vi "GIP CAN Wrapper.vi"(6 "Signal Write":dbl, 7 "States":T1, 8 "error in":errorcluster, 9 "Setting":T2={"Termination"=1, "Baud Rate"=125000, "Interface"="CAN1", "XNET Database"="can_messages_818", "ECU"="GIP\ncan_messages_818"} {"Termination" items=["Off", "On"]}, 10 "Tx Signal In":string="\"GIP_TestMode.GIP_TestModeFlag\"", 11 "Rx Signal In":string="\"GIP_Status.GIP_State\"") -> (0 "error out":errorcluster={"status"=TRUE, "code"=-1074384711, "source"="XNET Create Session (Signal Input Single-point).vi:6590001<APPEND>\n\n<b>Complete call chain:</b>\r\n     XNET Create Session (Signal Input Single-point).vi:6590001\r\n     CAN GIP.lvlib:GIP CAN Wrapper.vi"}, 1 "Tx Sigs":refnum<k21>[](array[refnum]), 2 "Rx Sigs":refnum<k21>[](array[refnum]), 3 "Signal out":dbl=nan)   [LabVIEW 2021, in "CAN GIP.lvlib"]
uses:
  CAN GIP.lvlib
  Private Controls/Setting.ctl
  Private Controls/CAN States.ctl
  Private Controls/Local Variables.ctl
  <vilib>/JDP Science/JSONtext/Next JSON Value.vi
  <vilib>/JDP Science/JSONtext/String Subset.vi
  <vilib>/JDP Science/JSONtext/Parsing/Advance past next JSON Value (inlined COPY).vi
  <vilib>/JDP Science/JSONtext/Parsing/Advance past whitespace.vi
  <vilib>/JDP Science/JSONtext/Parsing/Advance past String.vi
  <vilib>/JDP Science/JSONtext/Parsing/Advance past Number.vi
  <vilib>/JDP Science/JSONtext/Parsing/Advance past Line Ending.vi
  <vilib>/xnet/xnet.llb/XNET Create Session (Signal Input Single-point).vi
  <vilib>/xnet/xnet.llb/XNET Create Session (Signal Output Single-point).vi
  <vilib>/xnet/xnet.llb/XNET Read (Signal Single-point).vi
  <vilib>/JDP Science/JSONtext/Parsing/Parse Full Path or Item Name.vi
  <vilib>/JDP Science/JSONtext/Parsing/Advance past Array.vi
  <vilib>/JDP Science/JSONtext/Parsing/Advance past Object.vi
  <vilib>/JDP Science/JSONtext/support/Error Cluster From Code.vi
  <vilib>/JDP Science/JSONtext/Offset/Find Item Locations by Path.vi
  <vilib>/xnet/xnet.llb/XNET Write (Signal Single-point).vi
  <resource>/objmgr/xnet.rc
  <vilib>/JDP Science/JSONtext/JSONtext.lvlib
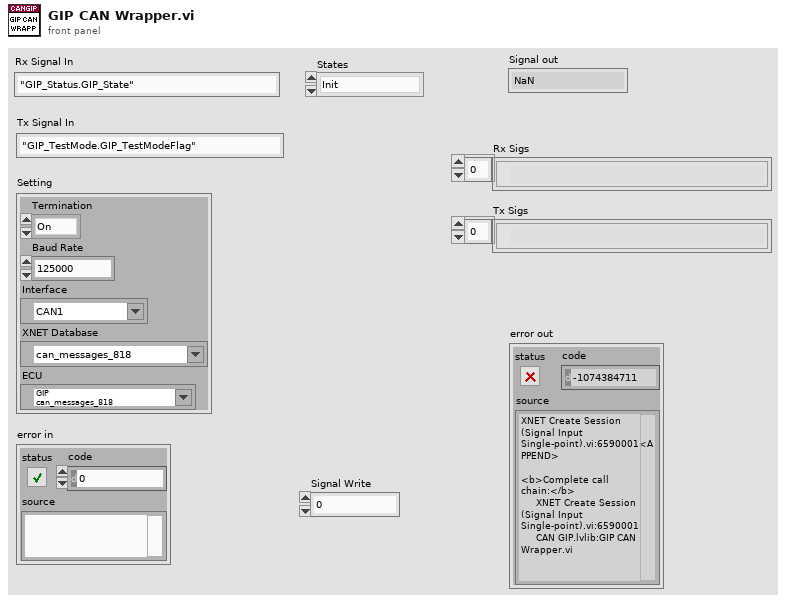
[diagram p1: front panel]
types:
  T1 = typedef "CAN GIP.lvlib/CAN States.ctl" = enum16{"Init", "Config", "Read Signals", "Write Signals", "Close"}
  T2 = typedef "CAN GIP.lvlib/Setting.ctl" = cluster{"Termination":u32, "Baud Rate":u64, "Interface":refnum<k21>, "XNET Database":refnum<k21>, "ECU":refnum<k21>}
  T3 = typedef "CAN GIP.lvlib/Local Variables.ctl" = cluster{"Rx session":refnum<k21>, "Tx session":refnum<k21>, "Tx Data":dbl[], "JSON":string}
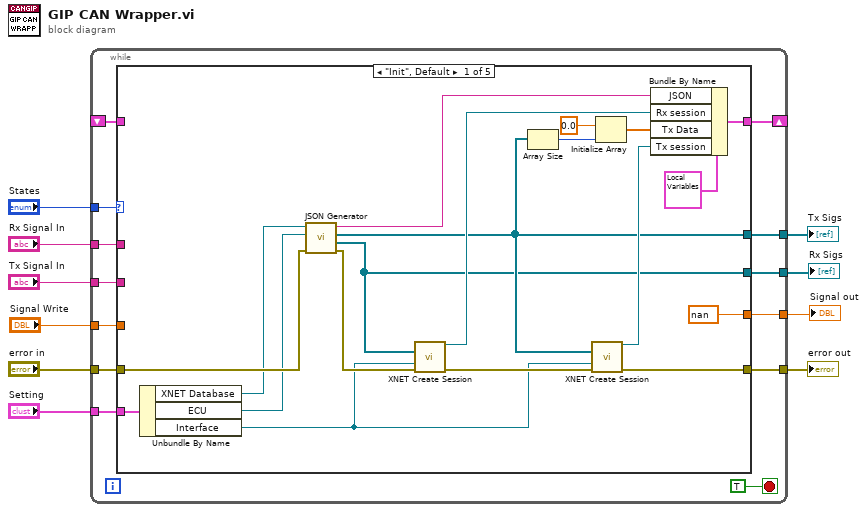
[diagram p0: block diagram]
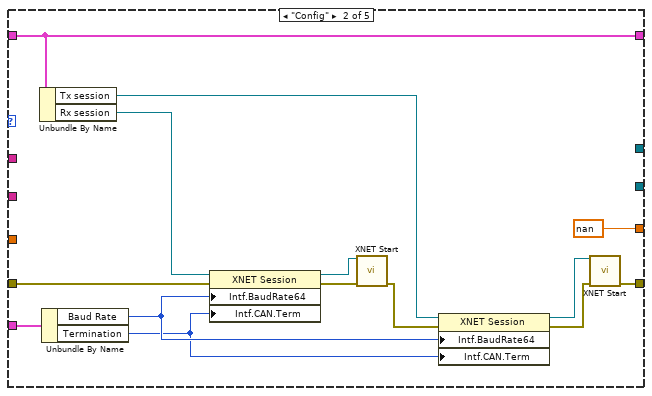
[diagram p2: hidden frame]
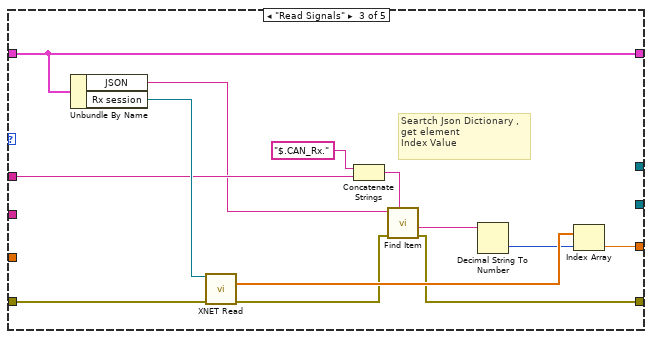
[diagram p3: hidden frame]
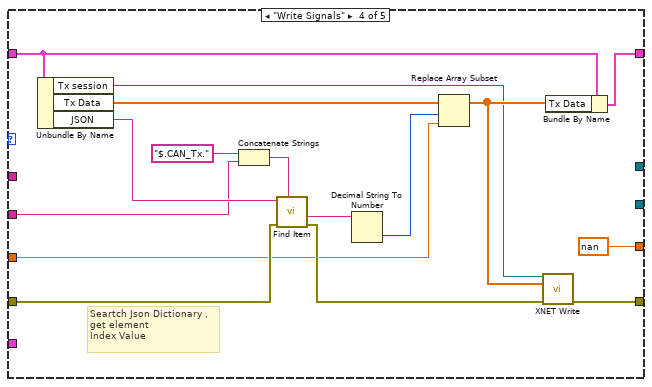
[diagram p4: hidden frame]
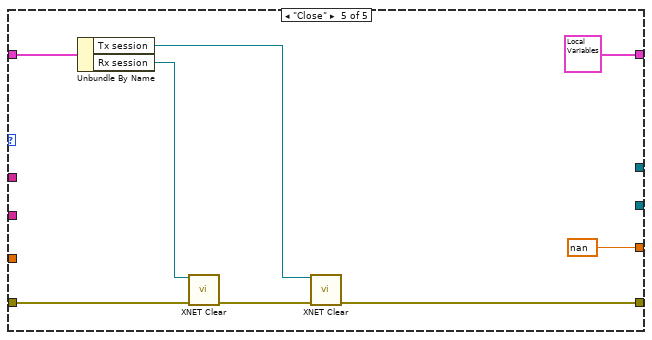
[diagram p5: hidden frame]
diagram:
  n1 = while {
    tunnel: "States" -> [w22]
    tunnel: "error in" -> [w21]
    tunnel: [w20] -> w9
    shift-right: [w19] -> _
    shift-left: _ -> [w18]
    tunnel: "Setting" -> [w17]
    tunnel: "Rx Signal In" -> [w16]
    tunnel: [w15] -> w5
    tunnel: "Signal Write" -> [w14]
    tunnel: "Tx Signal In" -> [w13]
    tunnel: [w12] -> w2
    tunnel: [w11] -> w1
    stop <- TRUE stop-if-true
    n2 = case shown="\"Init\", Default" w22 {
      tunnel: w21 -> [w33 w50 w69 w78 w93]
      tunnel: [w38 w46 w59 w85 w90] -> w20
      tunnel: [w41 w54 w67 w71 T3 {"Rx session"="", "Tx session"="", "Tx Data"=[], "JSON"="{\n  \"CAN_Rx\":{\n    \"GIP_GetPartNumber.lChar0\":0,\n    \"GIP_GetPartNumber.lChar1\":1,\n    \"GIP_GetPartNumber.lChar2\":2,\n    \"GIP_GetPartNumber.lChar3\":3,\n    \"GIP_GetPartNumber.lChar4\":4,\n    \"GIP_GetPartNumber.lChar5\":5,\n    \"GIP_GetPartNumber.lChar6\":6,\n    \"GIP_GetPartNumber.lChar7\":7,\n    \"GIP_GetPartNumber.rChar0\":8,\n    \"GIP_GetPartNumber.rChar1\":9,\n    \"GIP_GetSerialNumber.vendorChar0\":10,\n    \"GIP_GetSerialNumber.vendorChar1\":11,\n    \"GIP_GetSerialNumber.vendorChar2\":12,\n    \"GIP_GetSerialNumber.weekAndSerial\":13,\n    \"GIP_Grid_ActiveEnergyExported.GIP_Grid_ActiveEnergyExported_L1\":14,\n    \"GIP_Grid_ActiveEnergyExported.GIP_Grid_ActiveEnergyExported_L2\":15,\n    \"GIP_Grid_ActiveEnergyImported.GIP_Grid_ActiveEnergyImported_L1\":16,\n    \"GIP_Grid_ActiveEnergyImported.GIP_Grid_ActiveEnergyImported_L2\":17,\n    \"GIP_Grid_Power.GIP_Grid_ActivePower_L1\":18,\n    \"GIP_Grid_Power.GIP_Grid_ActivePower_L2\":19,\n    \"GIP_Grid_Power.GIP_Grid_ReactivePower_L1\":20,\n    \"GIP_Grid_Power.GIP_Grid_ReactivePower_L2\":21,\n    \"GIP_Grid_TotalActiveEnergy.GIP_Grid_TotalActiveEnergyExported\":22,\n    \"GIP_Grid_TotalActiveEnergy.GIP_Grid_TotalActiveEnergyImported\":23,\n    \"GIP_Load_ActiveEnergyExported.GIP_Load_ActiveEnergyExported_L1\":24,\n    \"GIP_Load_ActiveEnergyExported.GIP_Load_ActiveEnergyExported_L2\":25,\n    \"GIP_Load_ActiveEnergyImported.GIP_Load_ActiveEnergyImported_L1\":26,\n    \"GIP_Load_ActiveEnergyImported.GIP_Load_ActiveEnergyImported_L2\":27,\n    \"GIP_Load_Power.GIP_Load_ActivePower_L1\":28,\n    \"GIP_Load_Power.GIP_Load_ActivePower_L2\":29,\n    \"GIP_Load_Power.GIP_Load_ReactivePower_L1\":30,\n    \"GIP_Load_Power.GIP_Load_ReactivePower_L2\":31,\n    \"GIP_Load_TotalActiveEnergy.GIP_Load_TotalActiveEnergyExported\":32,\n    \"GIP_Load_TotalActiveEnergy.GIP_Load_TotalActiveEnergyImported\":33,\n    \"GIP_Status.GIP_Relay_State\":34,\n    \"GIP_Status.GIP_State\":35\n  },\n  \"CAN_Tx\":{\n    \"GIP_ManufacturingControl.ESP32Comms\":0,\n    \"GIP_ManufacturingControl.FaultLED\":1,\n    \"GIP_ManufacturingControl.Relay\":2,\n    \"GIP_ManufacturingControl.ST8500Comms\":3,\n    \"GIP_ManufacturingControl.StatusLED\":4,\n    \"GIP_SetPartNumber.lChar0\":5,\n    \"GIP_SetPartNumber.lChar1\":6,\n    \"GIP_SetPartNumber.lChar2\":7,\n    \"GIP_SetPartNumber.lChar3\":8,\n    \"GIP_SetPartNumber.lChar4\":9,\n    \"GIP_SetPartNumber.lChar5\":10,\n    \"GIP_SetPartNumber.lChar6\":11,\n    \"GIP_SetPartNumber.lChar7\":12,\n    \"GIP_SetPartNumber.rChar0\":13,\n    \"GIP_SetPartNumber.rChar1\":14,\n    \"GIP_SetSerialNumber.vendorChar0\":15,\n    \"GIP_SetSerialNumber.vendorChar1\":16,\n    \"GIP_SetSerialNumber.vendorChar2\":17,\n    \"GIP_SetSerialNumber.weekAndSerial\":18,\n    \"GIP_SetTestedFlag.GIP_TestedFlag\":19,\n    \"GIP_TestMode.GIP_TestModeFlag\":20\n  }\n}"}] -> w19
      tunnel: w18 -> [_ w54 w67 w74 w92]
      tunnel: w17 -> [w29 w55 _ _ _]
      tunnel: w16 -> [_ _ w62 _ _]
      tunnel: [nan nan w65 nan nan] -> w15
      tunnel: w14 -> [_ _ _ w76 _]
      tunnel: w13 -> [_ _ _ w75 _]
      tunnel: [w25 _ _ _ _] -> w12
      tunnel: [w24 _ _ _ _] -> w11
      frame "Init", Default {
        n3 = Unbundle By Name(w29) -> ("XNET Database"=w28:refnum<k21>, "ECU"=w27:refnum<k21>, "Interface"=w26:refnum<k21>)
        n4 = call "JSON Generator.vi"("error in (no error)"=w33, "ECU"=w27, "XNET Database"=w28) -> ("error out"=w32:errorcluster, "Rx Sigs"=w24:refnum<k21>[], "Tx Sigs"=w25:refnum<k21>[], "JSON"=w31:string)  [unwired: 5 in]
        n5 = call-poly <vilib>:"XNET Create Session.vi"("signal list"=w24, "interface"=w26, "error in (no error)"=w32) -> ("session out"=w39:refnum<k21>, "error out"=w40:errorcluster)  [unwired: 11 out]
        n6 = Array Size(array=w25) -> (size(s)=w37:i32)
        n7 = call-poly <vilib>:"XNET Create Session.vi"("signal list"=w25, "interface"=w26, "error in (no error)"=w40) -> ("session out"=w30:refnum<k21>, "error out"=w38:errorcluster)  [unwired: 11 out]
        n8 = Initialize Array(0.0 ("element"), w37) -> (w35:dbl[])
        n9 = Bundle By Name(cluster=T3 {"Rx session"="", "Tx session"="", "Tx Data"=[], "JSON"="{\n  \"CAN_Rx\":{\n    \"GIP_GetPartNumber.lChar0\":0,\n    \"GIP_GetPartNumber.lChar1\":1,\n    \"GIP_GetPartNumber.lChar2\":2,\n    \"GIP_GetPartNumber.lChar3\":3,\n    \"GIP_GetPartNumber.lChar4\":4,\n    \"GIP_GetPartNumber.lChar5\":5,\n    \"GIP_GetPartNumber.lChar6\":6,\n    \"GIP_GetPartNumber.lChar7\":7,\n    \"GIP_GetPartNumber.rChar0\":8,\n    \"GIP_GetPartNumber.rChar1\":9,\n    \"GIP_GetSerialNumber.vendorChar0\":10,\n    \"GIP_GetSerialNumber.vendorChar1\":11,\n    \"GIP_GetSerialNumber.vendorChar2\":12,\n    \"GIP_GetSerialNumber.weekAndSerial\":13,\n    \"GIP_Grid_ActiveEnergyExported.GIP_Grid_ActiveEnergyExported_L1\":14,\n    \"GIP_Grid_ActiveEnergyExported.GIP_Grid_ActiveEnergyExported_L2\":15,\n    \"GIP_Grid_ActiveEnergyImported.GIP_Grid_ActiveEnergyImported_L1\":16,\n    \"GIP_Grid_ActiveEnergyImported.GIP_Grid_ActiveEnergyImported_L2\":17,\n    \"GIP_Grid_Power.GIP_Grid_ActivePower_L1\":18,\n    \"GIP_Grid_Power.GIP_Grid_ActivePower_L2\":19,\n    \"GIP_Grid_Power.GIP_Grid_ReactivePower_L1\":20,\n    \"GIP_Grid_Power.GIP_Grid_ReactivePower_L2\":21,\n    \"GIP_Grid_TotalActiveEnergy.GIP_Grid_TotalActiveEnergyExported\":22,\n    \"GIP_Grid_TotalActiveEnergy.GIP_Grid_TotalActiveEnergyImported\":23,\n    \"GIP_Load_ActiveEnergyExported.GIP_Load_ActiveEnergyExported_L1\":24,\n    \"GIP_Load_ActiveEnergyExported.GIP_Load_ActiveEnergyExported_L2\":25,\n    \"GIP_Load_ActiveEnergyImported.GIP_Load_ActiveEnergyImported_L1\":26,\n    \"GIP_Load_ActiveEnergyImported.GIP_Load_ActiveEnergyImported_L2\":27,\n    \"GIP_Load_Power.GIP_Load_ActivePower_L1\":28,\n    \"GIP_Load_Power.GIP_Load_ActivePower_L2\":29,\n    \"GIP_Load_Power.GIP_Load_ReactivePower_L1\":30,\n    \"GIP_Load_Power.GIP_Load_ReactivePower_L2\":31,\n    \"GIP_Load_TotalActiveEnergy.GIP_Load_TotalActiveEnergyExported\":32,\n    \"GIP_Load_TotalActiveEnergy.GIP_Load_TotalActiveEnergyImported\":33,\n    \"GIP_Status.GIP_Relay_State\":34,\n    \"GIP_Status.GIP_State\":35\n  },\n  \"CAN_Tx\":{\n    \"GIP_ManufacturingControl.ESP32Comms\":0,\n    \"GIP_ManufacturingControl.FaultLED\":1,\n    \"GIP_ManufacturingControl.Relay\":2,\n    \"GIP_ManufacturingControl.ST8500Comms\":3,\n    \"GIP_ManufacturingControl.StatusLED\":4,\n    \"GIP_SetPartNumber.lChar0\":5,\n    \"GIP_SetPartNumber.lChar1\":6,\n    \"GIP_SetPartNumber.lChar2\":7,\n    \"GIP_SetPartNumber.lChar3\":8,\n    \"GIP_SetPartNumber.lChar4\":9,\n    \"GIP_SetPartNumber.lChar5\":10,\n    \"GIP_SetPartNumber.lChar6\":11,\n    \"GIP_SetPartNumber.lChar7\":12,\n    \"GIP_SetPartNumber.rChar0\":13,\n    \"GIP_SetPartNumber.rChar1\":14,\n    \"GIP_SetSerialNumber.vendorChar0\":15,\n    \"GIP_SetSerialNumber.vendorChar1\":16,\n    \"GIP_SetSerialNumber.vendorChar2\":17,\n    \"GIP_SetSerialNumber.weekAndSerial\":18,\n    \"GIP_SetTestedFlag.GIP_TestedFlag\":19,\n    \"GIP_TestMode.GIP_TestModeFlag\":20\n  }\n}"}, "JSON"=w31, "Rx session"=w39, "Tx Data"=w35, "Tx session"=w30) -> (w41:T3)
      }
      frame "Config" {
        n10 = Unbundle By Name(w54) -> ("Tx session"=w53:refnum<k21>, "Rx session"=w56:refnum<k21>)
        n11 = Unbundle By Name(w55) -> ("Baud Rate"=w52:u64, "Termination"=w51:u32)
        n12 = property class="XNET Session"(reference=w56, error in=w50, "Intf.BaudRate64"=w52, "Intf.CAN.Term"=w51) -> (reference out=w47:refnum<k21>, error out=w49:errorcluster)
        n13 = call <vilib>:"XNET Start.vi"("session in"=w47, "error in (no error)"=w49) -> ("error out"=w48:errorcluster)  [unwired: 12 in, 1 out]
        n14 = property class="XNET Session"(reference=w53, error in=w48, "Intf.BaudRate64"=w52, "Intf.CAN.Term"=w51) -> (reference out=w44:refnum<k21>, error out=w45:errorcluster)
        n15 = call <vilib>:"XNET Start.vi"("session in"=w44, "error in (no error)"=w45) -> ("error out"=w46:errorcluster)  [unwired: 12 in, 1 out]
      }
      frame "Read Signals" {
        # "Seartch Json Dictionary ,\nget element\nIndex Value"
        n16 = Unbundle By Name(w67) -> ("JSON"=w61:string, "Rx session"=w68:refnum<k21>)
        n17 = call-poly <vilib>:"XNET Read.vi"("session in"=w68, "error in (no error)"=w69) -> ("data"=w66:dbl[], "error out"=w60:errorcluster)  [unwired: 12 out]
        n18 = Concatenate Strings("$.CAN_Rx." ("$Path or Item Name"), w62) -> (w63:string)
        n19 = call <vilib>:"Find Item.vi"("$Path or Item Name"=w63, "error in (no error)"=w60, "JSON"=w61) -> ("error out"=w59:errorcluster, "<JSON>"=w57:string)  [unwired: 5 in, 2 out]
        n20 = Decimal String To Number(string=w57) -> (number=w58:i32)  [unwired: 2 in, 1 out]
        n21 = Index Array(array=w66, index=w58) -> (element=w65:dbl)
      }
      frame "Write Signals" {
        # "Seartch Json Dictionary ,\nget element\nIndex Value"
        n22 = Unbundle By Name(w74) -> ("Tx session"=w70:refnum<k21>, "Tx Data"=w73:dbl[], "JSON"=w80:string)
        n23 = Concatenate Strings("$.CAN_Tx." ("$Path or Item Name"), w75) -> (w81:string)
        n24 = call <vilib>:"Find Item.vi"("$Path or Item Name"=w81, "error in (no error)"=w78, "JSON"=w80) -> ("error out"=w77:errorcluster, "<JSON>"=w83:string)  [unwired: 5 in, 2 out]
        n25 = Decimal String To Number(string=w83) -> (number=w79:i32)  [unwired: 2 in, 1 out]
        n26 = Replace Array Subset(array=w73, new element=w76, index=w79) -> (w72:dbl[])
        n27 = call-poly <vilib>:"XNET Write.vi"("session in"=w70, "data"=w72, "error in (no error)"=w77) -> ("error out"=w85:errorcluster)  [unwired: 12 out]
        n28 = Bundle By Name(cluster=w74, "Tx Data"=w72) -> (w71:T3)
      }
      frame "Close" {
        n29 = Unbundle By Name(w92) -> ("Tx session"=w88:refnum<k21>, "Rx session"=w89:refnum<k21>)
        n30 = call <vilib>:"XNET Clear.vi"("session in"=w89, "error in (no error)"=w93) -> ("error out"=w91:errorcluster)  [unwired: 13 in]
        n31 = call <vilib>:"XNET Clear.vi"("session in"=w88, "error in (no error)"=w91) -> ("error out"=w90:errorcluster)  [unwired: 13 in]
      }
    }
  }
  "error out" <- w9
  "Signal out" <- w5
  "Tx Sigs" <- w2
  "Rx Sigs" <- w1
